vi "Write TC State Machine Setups.vi"(4 "Error In":errorcluster, 5 "TC Parameters":T1, 6 "Instance Name":T2, 7 "Config Data_DB_ADO in":refnum<class "Config Data_DB_ADO.lvclass">) -> (0 "Error Out":errorcluster, 3 "Config Data_DB_ADO out":refnum<class "Config Data_DB_ADO.lvclass">)   [LabVIEW 2020, in "Config Data.lvlib" / "Config Data_DB_ADO.lvclass"]
uses:
  Config Data_DB_ADO.lvclass
  toolbox/ADO Database Drivers/ADO Database Drivers.lvlib
  Config Data_DB.lvclass
  C:/Users/Fred Guo/Desktop/Release 19/_libraries/Config Data/DB/Config Data_DB.lvclass
  C:/Users/Fred Guo/Desktop/Release 19/_libraries/Config Data/Config Data.lvclass
  C:/Users/Fred Guo/Desktop/Release 19/_libraries/Config Data/DB/ADO/Config Data_DB_ADO.lvclass
  Startup Processes/_typedefs/Subpanel Names.ctl
  Startup Processes/Startup Processes.lvlib
  Startup Processes/_typedefs/TC Setup Parameters.ctl
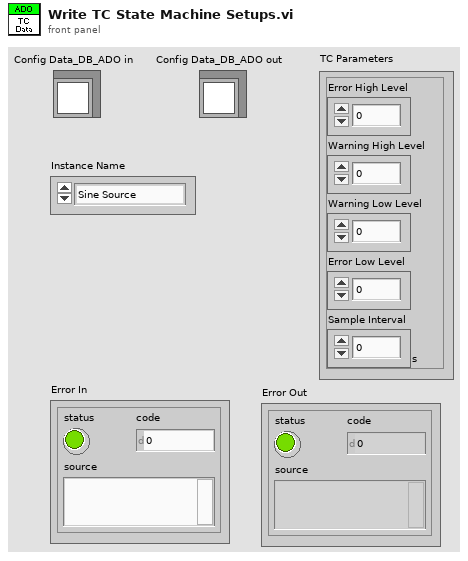
[diagram p1: front panel]
types:
  T1 = typedef "Startup Processes.lvlib/TC Setup Parameters.ctl" = cluster{"Error High Level":dbl, "Warning High Level":dbl, "Warning Low Level":dbl, "Error Low Level":dbl, "Sample Interval":dbl[unit]}
  T2 = typedef "Startup Processes.lvlib/Subpanel Names.ctl" = enum16{"Sine Source", "Ramp Source", "Hen House TC", "Dog House TC", "Out House TC"}
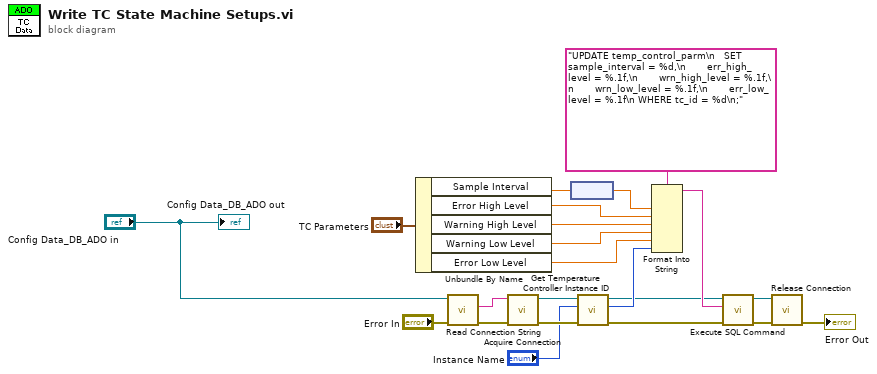
[diagram p0: block diagram]
diagram:
  n1 = Unbundle By Name("TC Parameters") -> ("Sample Interval"=w3:dbl[unit], "Error High Level"=w4:dbl, "Warning High Level"=w6:dbl, "Warning Low Level"=w5:dbl, "Error Low Level"=w2:dbl)
  n2 = call "Read Connection String.vi"("Error In"="Error In", "DB In"="Config Data_DB_ADO in") -> ("Error Out"=w11:errorcluster, "Connection String"=w10:string)  [unwired: 3 in, 1 out]
  n3 = call "Acquire Connection.vi"("error in (no error)"=w11, "Connection String"=w10) -> ("error out"=w13:errorcluster, "Connection"=w12:refnum<k7>)  [unwired: 3 in, 1 out]
  n4 = node(w3) -> (w1:dbl)
  n5 = call "Get Temperature Controller Instance ID.vi"("error in (no error)"=w13, "Instance Name"="Instance Name", "Connection In"=w12) -> ("error out"=w16:errorcluster, "tc_id"=w15:i32, "Connection Out"=w14:refnum<k7>)  [unwired: 2 in]
  n6 = Format Into String(format string="UPDATE temp_control_parm\n   SET sample_interval = %d,\n       err_high_level = %.1f,\n       wrn_high_level = %.1f,\n       wrn_low_level = %.1f,\n       err_low_level = %.1f\n WHERE tc_id = %d\n;", w1, w4, w6, w5, w2, w15) -> (resulting string=w18:string)  [unwired: 2 in, 1 out]
  n7 = call "Execute SQL Command.vi"("error in"=w16, "SQL Command"=w18, "Connection In"=w14) -> ("error out"=w20:errorcluster, "Connection Out"=w19:refnum<k7>)  [unwired: 2 in, 1 out]
  n8 = call "Release Connection.vi"("error in"=w20, "Connection"=w19) -> ("error out"=→"Error Out":errorcluster)  [unwired: 5 in]
  "Config Data_DB_ADO out" <- "Config Data_DB_ADO in"
